vi "PlotBoat.vi"(6 "Heading":dbl, 7 "Trace Path":bool=TRUE, 9 "MapDistanceInfo":T1 {"Top Left Pixel UTM"."North" format="%#_10f"; "Top Left Pixel UTM"."East" format="%#_8f"; "Bottom Right Pixel UTM"."North" format="%#_10f"; "Bottom Right Pixel UTM"."East" format="%#_8f"}, 10 "UTM Location":T2 {"North" format="%#_10f"; "East" format="%#_8f"}, 11 "Map in":T3) -> (2 "Boat Outside Img":bool, 3 "Map Out":T3)   [LabVIEW 2013]
uses:
  <vilib>/vision/Image Controls.llb/IMAQ Image.ctl
  cRIO_Code/Data/TypeDefs/UTM Location.ctl
  TypeDef/MapDistanceInfo.ctl
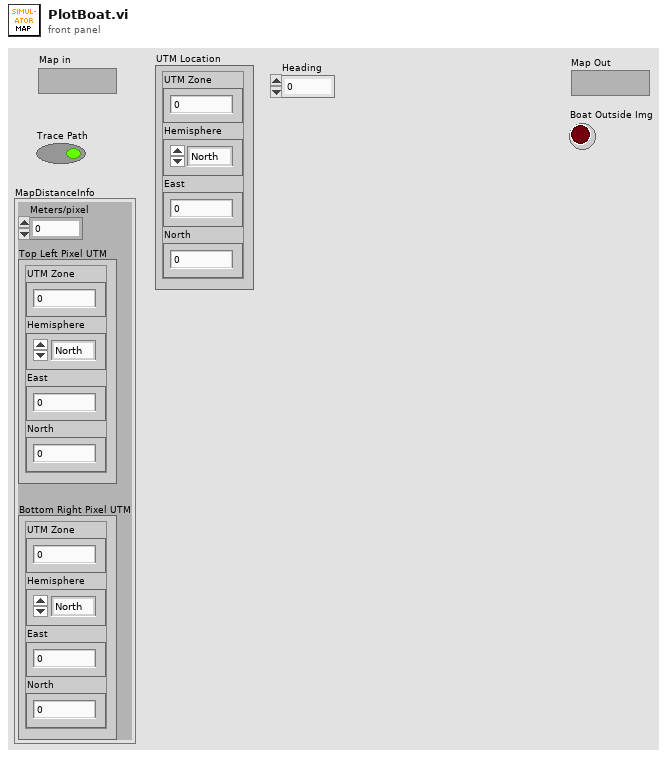
[diagram p1: front panel]
types:
  T1 = typedef "MapDistanceInfo.ctl" = cluster{"Meters/pixel":dbl, "Top Left Pixel UTM":T2, "Bottom Right Pixel UTM":T2}
  T2 = typedef "UTM Location.ctl" = cluster{"UTM Zone":dbl, "Hemisphere":enum16{"North", "South"}, "East":dbl, "North":dbl}
  T3 = typedef "IMAQ Image.ctl" = refnum<image>
  T4 = typedef "Overlay References.ctl" = cluster{"Boat Icon, Unroatated":T3, "Boat Icon, Rotated":T3, "Sail Icon, Unrotated":T3, "Sail Icon, Rotated":T3}
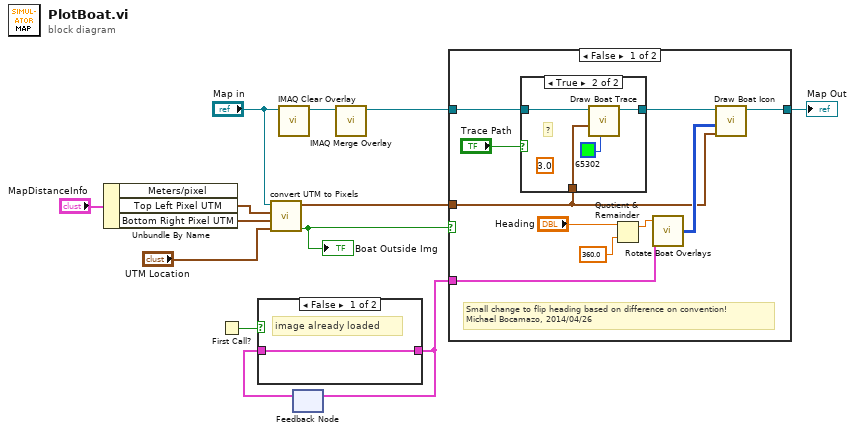
[diagram p0: block diagram]
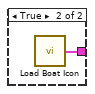
[diagram p4: hidden frame]
diagram:
  n1 = Unbundle By Name("MapDistanceInfo") -> ("Top Left Pixel UTM"=w2:T2, "Bottom Right Pixel UTM"=w1:T2)  [unwired: 1 out]
  n2 = First Call?() -> (First Call?: T/F=w12:bool)
  n3 = call "convert UTM to Pixels.vi"("UTM position of Boat"="UTM Location", "Bottum Right Pixel UTM"=w1, "Top Left Pixel UTM"=w2, "Map in"="Map in") -> ("Boat Outside Img"=w5:bool, "Position"=w4:cluster{"X":i32, "Y":i32})  [unwired: 6 in]
  "Boat Outside Img" <- w5
  n4 = call "IMAQ Clear Overlay"("Image"="Map in") -> ("Image Out"=w13:T3)  [unwired: 2 in, 8 out]
  n5 = feedback #1() -> (w10:T4)  [unwired: 1 in]
  n6 = case shown="False" w12 {
    tunnel: [w14 w15] -> w11
    tunnel: w10 -> [w14 _]
    frame False {
      # "image already loaded"
    }
    frame True {
      n7 = call "Load Boat Icon.vi"() -> ("Overlay References Out"=w15:T4)  [unwired: 1 in]
    }
  }
  n8 = feedback-in #1(w11) -> ()
  n9 = call "IMAQ Merge Overlay"("Image Src"=w13) -> ("Image Dst Out"=w9:T3)  [unwired: 4 in, 6 out]
  n10 = case shown="False" w5 {
    tunnel: [w23 w31] -> w8
    tunnel: w9 -> [w21 w31]
    tunnel: w11 -> [w24 _]
    tunnel: w4 -> [w20 _]
    frame False {
      # "Small change to flip heading based on difference on convention!\nMichael Bocamazo, 2014/04/26"
      n11 = case shown="True" "Trace Path" {
        tunnel: [w26 w29] -> w22
        tunnel: w21 -> [w26 w28]
        tunnel: w20 -> [_ w27]
        frame False {
        }
        frame True {
          (unwired) 3.0 ("Radius (px)")
          # "?"
          n12 = call "Draw Boat Trace.vi"("circle color"=u32 65302, "Position"=w27, "Image In"=w28) -> ("Image Out"=w29:T3)  [unwired: 8 in]
        }
      }
      n13 = Quotient & Remainder(x="Heading", y=360.0) -> (x-y*floor(x/y)=w18:dbl)  [unwired: 1 out]
      n14 = call "Rotate Boat Overlays.vi"("Overlay References In"=w24, "Heading"=w18) -> ("Rotated Boat Icon Bitmap Out"=w25:u32[][])  [unwired: 2 in, 1 out]
      n15 = call "Draw Boat Icon.vi"("Position"=w20, "Boat Bitmap"=w25, "Image In"=w22) -> ("Image Out"=w23:T3)  [unwired: 4 out]
    }
    frame True {
      # "don't draw\nif boat\noutside\nimage why not? lol"
    }
  }
  "Map Out" <- w8
